vi "Read Resolution Time.vi"(7 "Enum":T1, 8 "Error In":errorcluster, 11 "DVR IN":refnum<data-value>) -> (0 "Error Out":errorcluster, 1 "Surveys Count":i32, 2 "Average":dbl, 3 "Data Value Reference out":refnum<data-value>)   [LabVIEW 2016, in "Data Operations.lvlib"]
uses:
  Data Operations.lvlib
  Private Controls/Data Raw.ctl
  Private Controls/Survey Results Enum.ctl
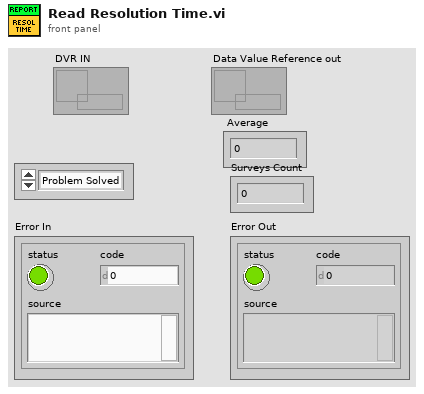
[diagram p1: front panel]
types:
  T1 = typedef "Data Operations.lvlib/Survey Results Enum.ctl" = enum16{"Problem Solved", "Resolution Time", "Total Satisfaction", "Courtesy", "Response Time"}
  T2 = typedef "Data Operations.lvlib/Data Raw.ctl" = cluster{"SR Number":string, "Status":string, "Summary":string, "AE Owner":string, "AE Group":string, "SurveyData":cluster{"Resolution Time":dbl, "Total Satisfaction":dbl, "Response Time":dbl, "Courtesy":dbl, "Problem Solved":dbl}, "Time Data":cluster{"Last Update Date":timestamp, "Request Date":timestamp, "Request week":u8}}
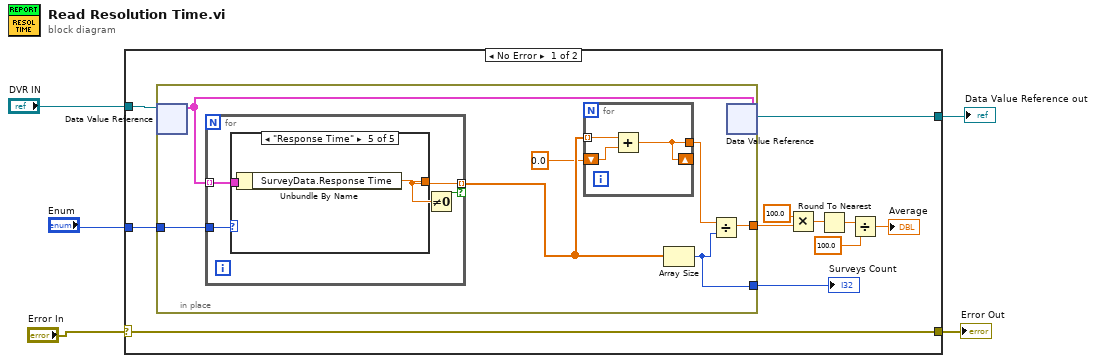
[diagram p0: block diagram]
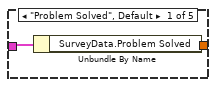
[diagram p2: hidden frame]
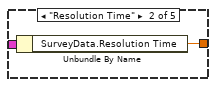
[diagram p3: hidden frame]
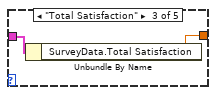
[diagram p4: hidden frame]
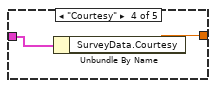
[diagram p5: hidden frame]
diagram:
  n1 = case shown="No Error" "Error In" {
    selector: "Error In" -> [w15 w42]
    tunnel: [w16 w41] -> w5
    tunnel: "DVR IN" -> [w6 w41]
    tunnel: [w15 w42] -> w2
    tunnel: "Enum" -> [w13 _]
    frame No Error {
      n2 = in-place {
        in-place-border: [w21] -> w12
        in-place-border: [w18] -> w14
        in-place-border: w13 -> [w17]
        n3 = in-place-dvr #1(w6) -> (w20:T2[])  [unwired: 1 out]
        n4 = for {
          tunnel: w20 -> [w27] mode=indexing
          tunnel: [w26] -> w23 mode=indexing if=w25
          tunnel: w17 -> [w24]
          n5 = case shown="\"Response Time\"" w24 {
            tunnel: w27 -> [w29 w31 w33 w35 w37]
            tunnel: [w28 w30 w32 w34 w36] -> w26
            frame "Problem Solved", Default {
              n6 = Unbundle By Name(w29) -> ("SurveyData.Problem Solved"=w28:dbl)
            }
            frame "Resolution Time" {
              n7 = Unbundle By Name(w31) -> ("SurveyData.Resolution Time"=w30:dbl)
            }
            frame "Total Satisfaction" {
              n8 = Unbundle By Name(w33) -> ("SurveyData.Total Satisfaction"=w32:dbl)
            }
            frame "Courtesy" {
              n9 = Unbundle By Name(w35) -> ("SurveyData.Courtesy"=w34:dbl)
            }
            frame "Response Time" {
              n10 = Unbundle By Name(w37) -> ("SurveyData.Response Time"=w36:dbl)
            }
          }
          n11 = Not Equal To 0?(x=w26) -> (x != 0?=w25:bool)
        }
        n12 = for {
          tunnel: w23 -> [w40] mode=indexing
          tunnel: [w38] -> w22
          shift-right: [w38] -> _
          shift-left: 0.0 -> [w39]
          n13 = Add(x=w40, y=w39) -> (x+y=w38:dbl)
        }
        n14 = Array Size(array=w23) -> (size(s)=w18:i32)
        n15 = Divide(x=w22, y=w18) -> (x/y=w21:dbl)
        n16 = in-place-dvr #1(w20) -> (w16:refnum<data-value>)  [unwired: 1 out]
      }
      "Surveys Count" <- w14
      n17 = Multiply(x=100.0, y=w12) -> (x*y=w10:dbl)
      n18 = Round To Nearest(number=w10) -> (nearest integer value=w9:dbl)
      n19 = Divide(x=w9, y=100.0) -> (x/y=→"Average":dbl)
    }
    frame Error {
    }
  }
  "Data Value Reference out" <- w5
  "Error Out" <- w2
